vi "SLM_Calibrator_MANUAL.vi"() -> ()   [LabVIEW 2022 SP3]
uses:
  <vilib>/Utility/error.llb/DialogType.ctl
panel:
  out "error out 2":errorcluster
  out "error out":errorcluster
  out "return value":T1={"x"=2592, "y"=1944, "FPS"=20.50524934383202, "Exposure"=70.26569}
  out "available cameras":cluster{string[], string[]}={["U3-368xXLE-M", "U3-38JxXLE-M"], ["4104401787", "4104527767"]}
  in  "Yoffset 2":dbl
  in  "Xoffset 2":dbl
  in  "Yoffset":dbl=-57.0
  in  "Xoffset":dbl=1306.0
  in  "wait time (s)":u32=2
  in  "Tab Control":enum32{"CCD plane", "Plot"}(tab)=enum."Plot"
  in  "FPS":dbl=20.50524934383202
  out "Image Out":T2(plugin-control)
  in  "Exposure":dbl=70.26569
  in  "Camera ID":u16(ring) caption="Camera" items=["U3-368xXLE-M", "U3-38JxXLE-M"]
  out "XY Graph":cluster{dbl, dbl}[](graph)
  out "45º":bool
  out "135º":bool=TRUE
  in  "Analizer":bool=TRUE
  in  "Gradient2":bool
  in  "Gradient1":bool
  out "Yi2":dbl=-234.1726618705036
  in  "Yc2":dbl(slide)=4.136690647482014 scale=0.0..10.0
  in  "Yf2:":dbl(slide)=5.467625899280575 scale=0.0..10.0
  out "Xi2":dbl=82.7639751552795
  in  "Xf2:":dbl(slide)=5.372670807453416 scale=0.0..10.0
  in  "Xc2":dbl(slide)=1.1180124223602483 scale=0.0..10.0
  out "CGH_y\nSLM2":T2(plugin-control)
  in  "Active1":bool=TRUE caption="Hide/Show (Show)"
  in  "Active2":bool=TRUE caption="Hide/Show (Show)"
  in  "STOP":bool caption="Stop (F)"
  out "PHASE":bool
  out "AMP":bool=TRUE
  in  "amp_phase":bool=TRUE
  out "SLM2 2":bool
  out "SLM1":bool=TRUE
  in  "SLMs":bool=TRUE
  in  "Folter to save:":string="IDSfirst"
  out "Images done":dbl(slide) scale=0.0..256.0
  out "Yi1":dbl=-61.63636363636361
  out "Xi1":dbl=1319.9969418960245
  in  "Yf1:":dbl(slide)=-2.1636363636363636 min=-5.0 max=5.0 scale=-5.0..5.0
  in  "Xf1:":dbl(slide)=0.20000000000000018 min=-5.0 max=5.0 scale=-5.0..5.0
  in  "Xc1":dbl(slide)=0.25993883792048944 scale=-5.0..5.0
  in  "Yc1":dbl(slide)=0.30909090909090864 scale=-5.0..5.0
  out "CGH_x\nSLM1":T2(plugin-control)
  in  "Ready?\nCalibrate!":bool caption="Stop (F)"
  # "X:"
  # "Y:"
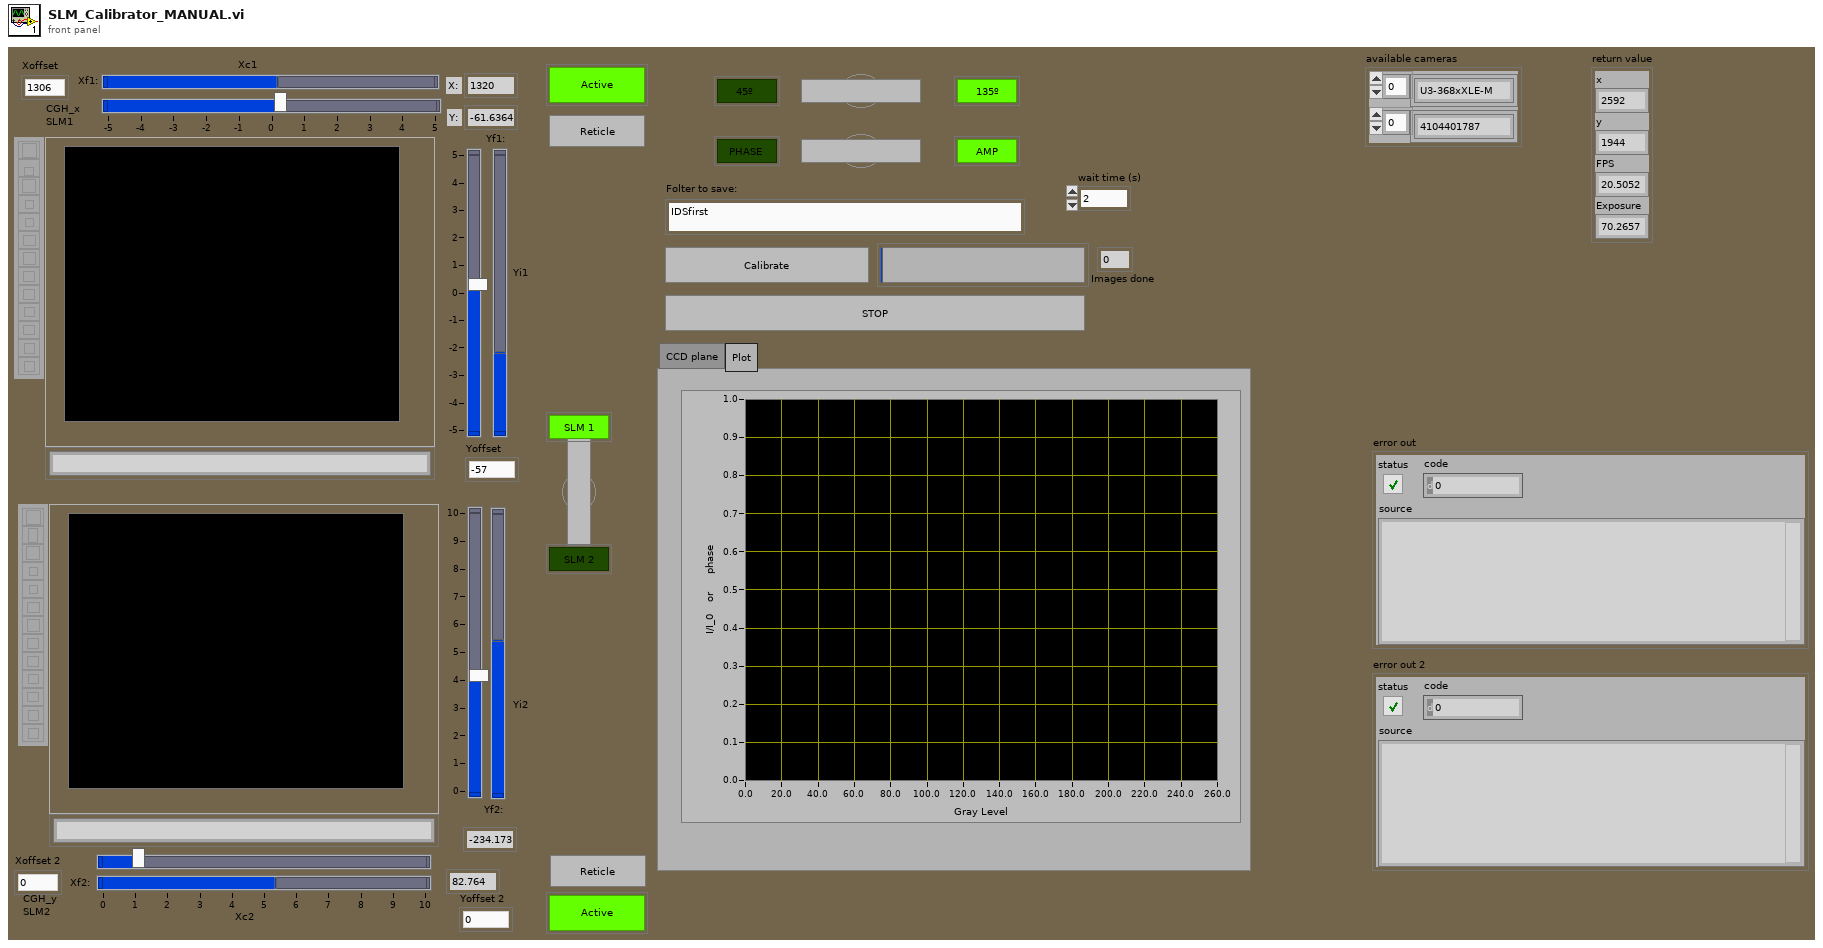
[diagram p1: front panel]
types:
  T1 = cluster{"x":i32, "y":i32, "FPS":dbl, "Exposure":dbl}
  T2 = typedef "IMAQ Image.ctl" = refnum<image>
  T3 = typedef "Image Type" = u32
  T4 = cluster{"Xoffset":dbl, "Yoffset":dbl, "Xc1":dbl, "Yc1":dbl, "Xf1:":dbl, "Yf1:":dbl}
  T5 = cluster{"Xoffset 2":dbl, "Yoffset 2":dbl, "Xc2":dbl, "Yc2":dbl, "Xf2:":dbl, "Yf2:":dbl}
  T6 = typedef "DialogType.ctl" = u16
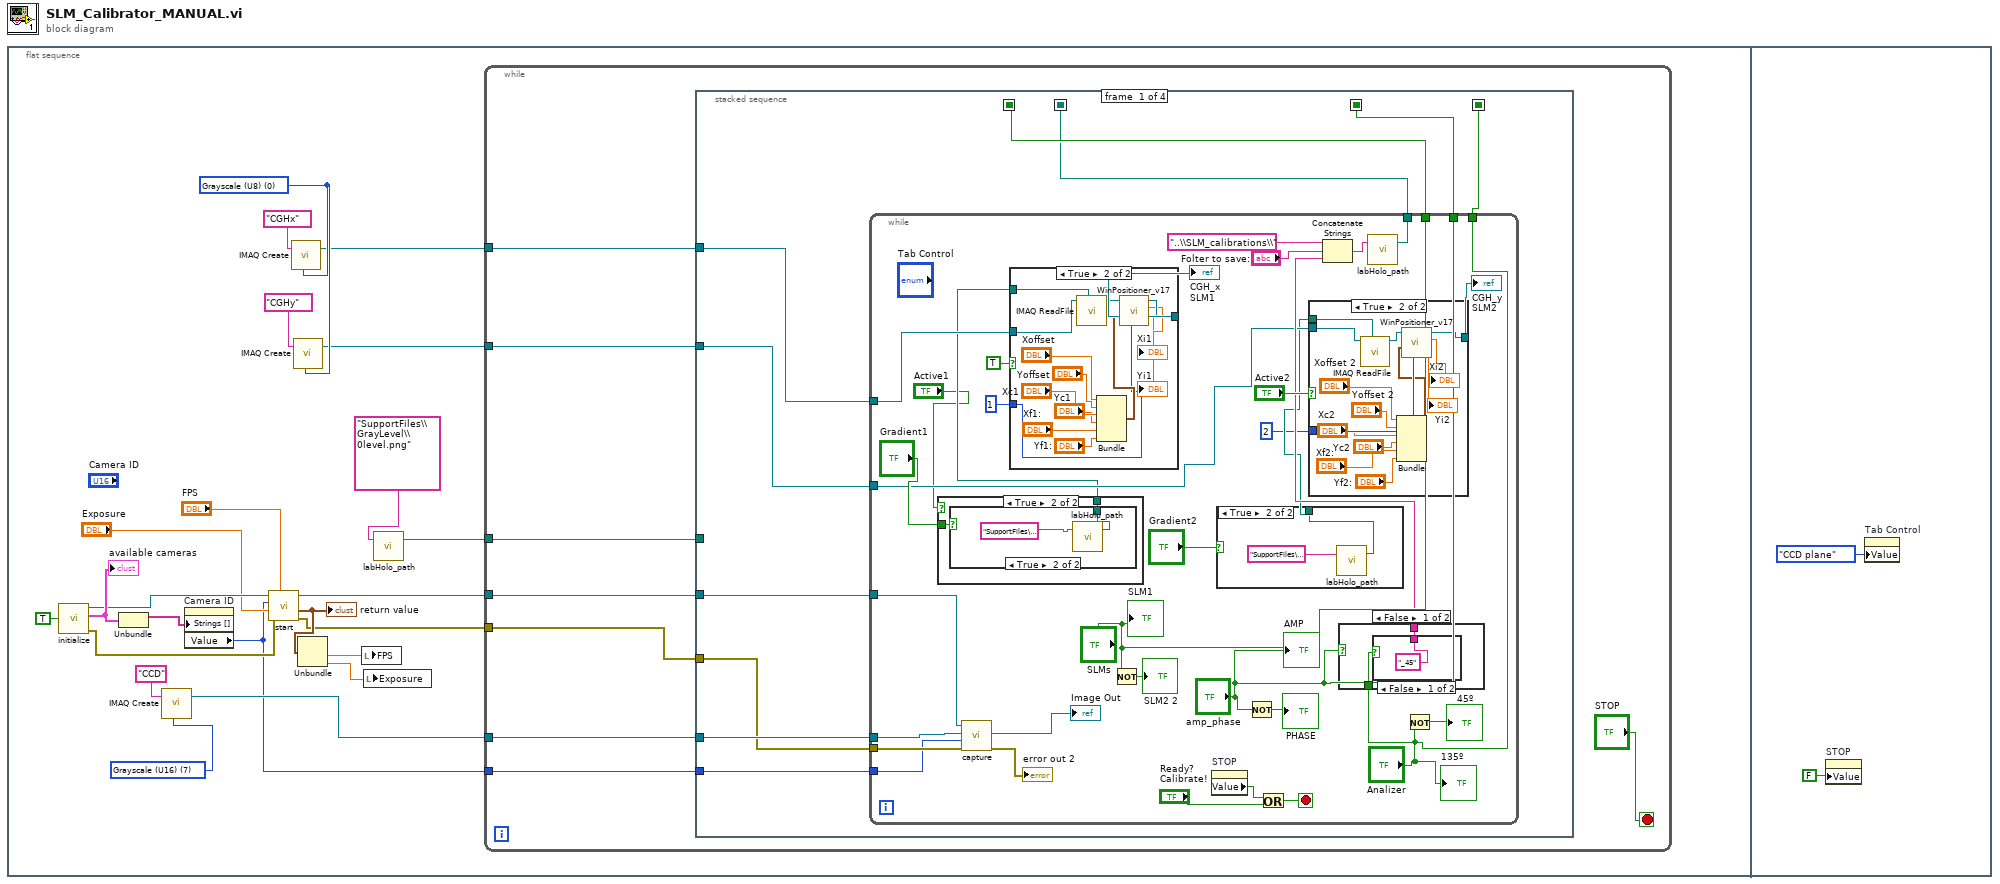
[diagram p0: block diagram]
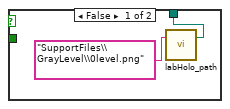
[diagram p2: hidden frame]
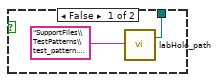
[diagram p3: hidden frame]
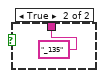
[diagram p4: hidden frame]
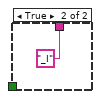
[diagram p5: hidden frame]
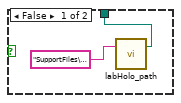
[diagram p6: hidden frame]
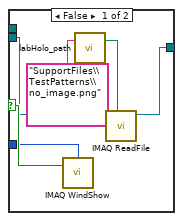
[diagram p7: hidden frame]
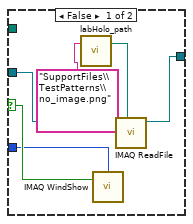
[diagram p8: hidden frame]
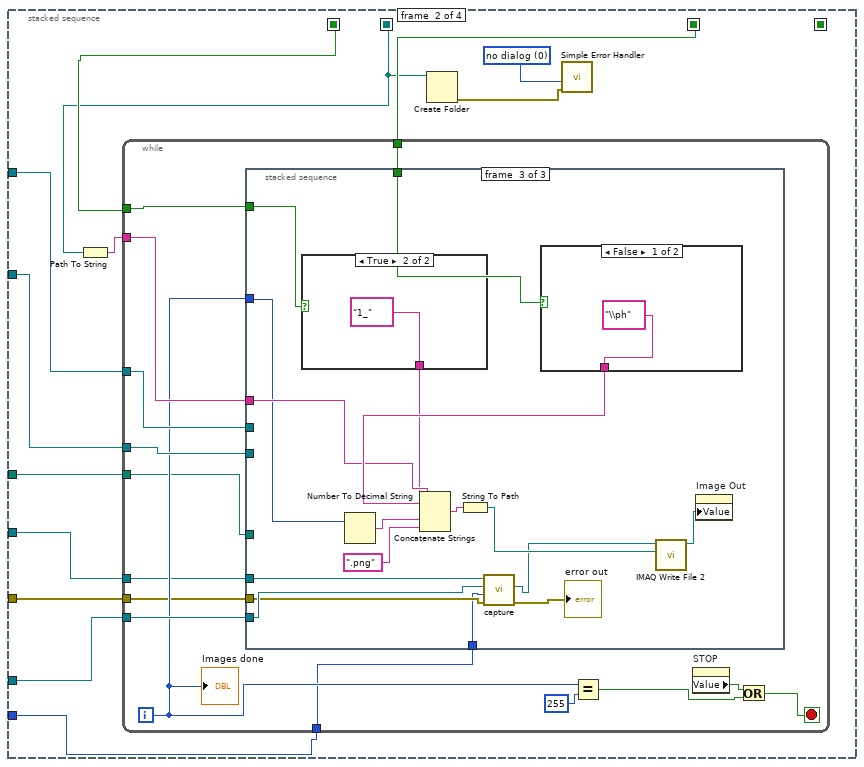
[diagram p9: hidden frame]
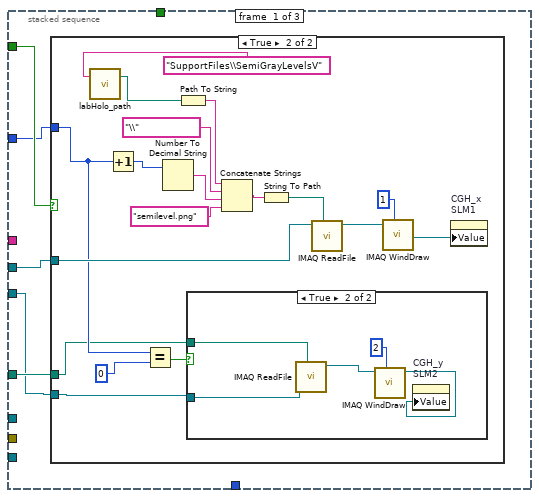
[diagram p10: hidden frame]
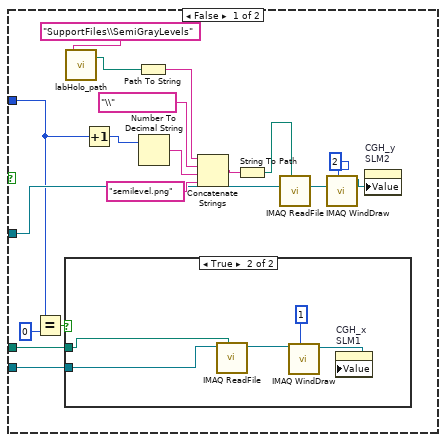
[diagram p11: hidden frame]
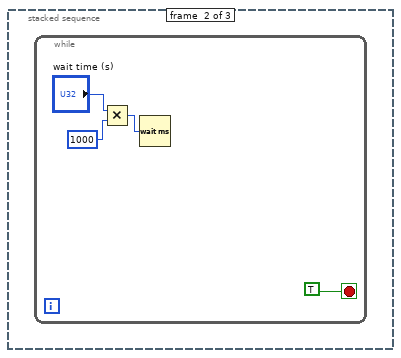
[diagram p14: hidden frame]
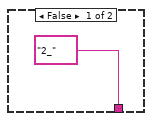
[diagram p15: hidden frame]
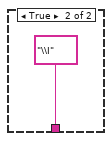
[diagram p16: hidden frame]
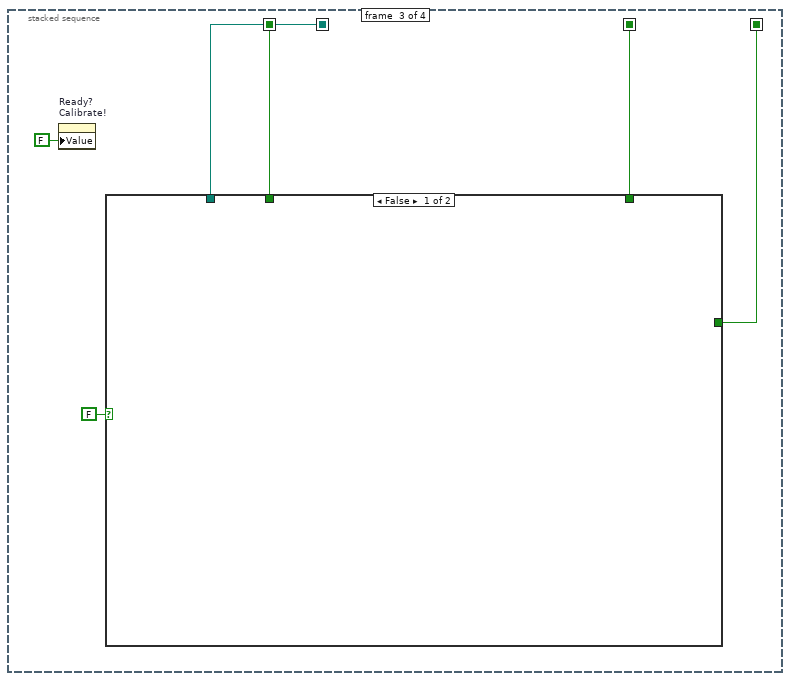
[diagram p17: hidden frame]
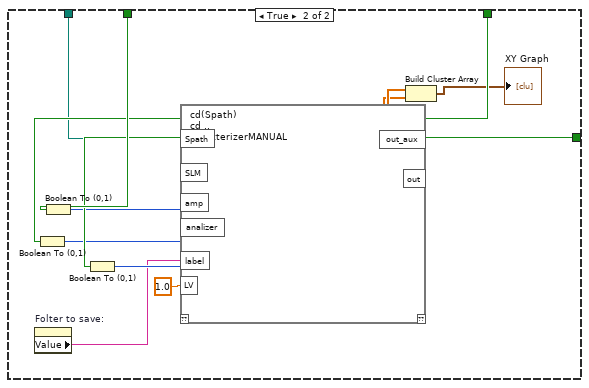
[diagram p18: hidden frame]
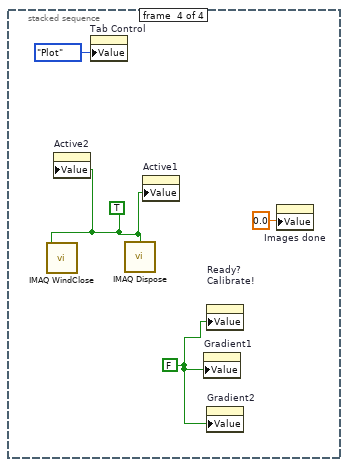
[diagram p19: hidden frame]
diagram:
  n1 = flat-sequence {
    frame #0 {
      w6 = T3 0 items=["Grayscale (U8)", "Grayscale (I16)", "Grayscale (SGL)", "Complex (CSG)", "RGB (U32)", "HSL (U32)", "RGB (U64)", "Grayscale (U16)"] ("Image Type")
      w21 = T3 7 items=["Grayscale (U8)", "Grayscale (I16)", "Grayscale (SGL)", "Complex (CSG)", "RGB (U32)", "HSL (U32)", "RGB (U64)", "Grayscale (U16)"] ("Image Type")
      n2 = call "initialize.vi"("14bits"=TRUE) -> ("session out"=w17:refnum<k35>, "available cameras"=w19:cluster{string[], string[]}, "error out"=w14:errorcluster)  [unwired: 3 in]
      "available cameras" <- w19
      n3 = Unbundle(w19) -> (w18:string[])  [unwired: 1 out]
      n4 = call "IMAQ Create"("Image Name"="CCD", "Image Type"=w21) -> ("New Image"=w20:T2)  [unwired: 3 in, 1 out]
      n5 = property on="Camera ID" class="Ring (strict)"("Strings []"=w18) -> ("Value"=w8:u16)  [unwired: 2 in, 2 out]
      n6 = call "start.vi"("FPS"="FPS", "error in (no error)"=w14, "Exposure (ms)"="Exposure", "Cam id"=w8, "session in"=w17) -> ("error out"=w9:errorcluster, "return value"=w13:T1, "session out"=w10:refnum<k35>)  [unwired: 2 in]
      "return value" <- w13
      n7 = call "IMAQ Create"("Image Name"="CGHx", "Image Type"=w6) -> ("New Image"=w3:T2)  [unwired: 3 in, 1 out]
      n8 = call "IMAQ Create"("Image Name"="CGHy", "Image Type"=w6) -> ("New Image"=w4:T2)  [unwired: 3 in, 1 out]
      n9 = Unbundle(w13) -> ("FPS"=w12:dbl, "Exposure"=w11:dbl)  [unwired: 2 out]
      n10 = local write "FPS"(w12) -> ()
      n11 = local write "Exposure"(w11) -> ()
      n12 = call "labHolo_path.vi"("sub folder or file (str)"="SupportFiles\\GrayLevel\\0level.png" ("name or relative path")) -> ("labHolo path"=w1:path)  [unwired: 1 in, 1 out]
      n13 = while {
        tunnel: w20 -> [w30]
        tunnel: w10 -> [w29]
        tunnel: w9 -> [w28]
        tunnel: w8 -> [w27]
        tunnel: w4 -> [w26]
        tunnel: w3 -> [w25]
        tunnel: w1 -> [w24]
        stop <- "STOP" stop-if-true
        n14 = stacked-sequence {
          seq-local: [w33 _ _ _] -> [_ w138 w239 _]
          seq-local: [w40 _ _ _] -> [_ w140 w241 _]
          seq-local: [w32 _ _ _] -> [_ w141 w240 _]
          seq-local: [w37 _ _ _] -> [_ _ w238 _]
          tunnel: w26 -> [w38 w143 _ _]
          tunnel: w25 -> [w39 w144 _ _]
          tunnel: w30 -> [w41 w139 _ _]
          tunnel: w29 -> [w36 w135 _ _]
          tunnel: w28 -> [w35 w134 _ _]
          tunnel: w27 -> [w34 w132 _ _]
          tunnel: w24 -> [_ w133 _ _]
          frame #0 {
            n15 = while {
              tunnel: w41 -> [w49]
              tunnel: [w42] -> w33
              tunnel: ["amp_phase"] -> w32
              tunnel: ["SLMs"] -> w40
              tunnel: w39 -> [w55]
              tunnel: w38 -> [w57]
              tunnel: ["Analizer"] -> w37
              tunnel: w36 -> [w47]
              tunnel: w35 -> [w46]
              tunnel: w34 -> [w45]
              stop <- w71 stop-if-true
              n16 = case shown="True" "Active1" {
                tunnel: "Gradient1" -> [_ w78]
                tunnel: [w75 w77] -> w54
                frame False {
                  n17 = call "labHolo_path.vi"("sub folder or file (str)"="SupportFiles\\GrayLevel\\0level.png" ("name or relative path")) -> ("labHolo path"=w75:path)  [unwired: 1 in, 1 out]
                }
                frame True {
                  n18 = case shown="True" w78 {
                    tunnel: [w79 w82] -> w77
                    frame False {
                      n19 = call "labHolo_path.vi"("sub folder or file (str)"="SupportFiles\\TestPatterns\\test_pattern.bmp" ("name or relative path")) -> ("labHolo path"=w79:path)  [unwired: 1 in, 1 out]
                    }
                    frame True {
                      n20 = call "labHolo_path.vi"("sub folder or file (str)"="SupportFiles\\TestPatterns\\test_pattern2V.png" ("name or relative path")) -> ("labHolo path"=w82:path)  [unwired: 1 in, 1 out]
                    }
                  }
                }
              }
              n21 = call "capture.vi"("error in (no error)"=w46, "Cam ID"=w45, "Image in"=w49, "session in"=w47) -> ("error out"=→"error out 2":errorcluster, "Image out"=→"Image Out":T2)  [unwired: 3 in, 1 out]
              n22 = case shown="True" TRUE {
                selector: TRUE -> [w117 _]
                tunnel: [w116 w128] -> w68
                tunnel: w55 -> [w115 w131]
                tunnel: w54 -> [_ w130]
                tunnel: 1 ("Window Number (0...15)") -> [w114 w118]
                frame False {
                  n23 = call "labHolo_path.vi"("sub folder or file (str)"="SupportFiles\\TestPatterns\\no_image.png" ("name or relative path")) -> ("labHolo path"=w112:path)  [unwired: 1 in, 1 out]
                  n24 = call "IMAQ WindShow"("Hide/Show (Show)"=w117, "Window Number (0...15)"=w114) -> ()  [unwired: 4 in, 3 out]
                  n25 = call "IMAQ ReadFile"("File Path"=w112, "Image"=w115) -> ("Image Out"=w116:T2)  [unwired: 5 in, 4 out]
                }
                frame True {
                  n26 = call "IMAQ ReadFile"("File Path"=w130, "Image"=w131) -> ("Image Out"=w129:T2)  [unwired: 5 in, 4 out]
                  n27 = Bundle("Xoffset"="Xoffset", "Yoffset"="Yoffset", "Xc1"="Xc1", "Yc1"="Yc1", "Xf1:"="Xf1:", "Yf1:"="Yf1:") -> (w125:T4)  [unwired: 1 in]
                  n28 = call "WinPositioner_v17.vi"("Display (1, 2...)"=w118, "Cluster"=w125, "Image"=w129) -> ("Y position"=→"Yi1":dbl, "X position"=→"Xi1":dbl, "CGH_x"=w128:T2)  [unwired: 6 in]
                }
              }
              "CGH_x\nSLM1" <- w68
              n29 = Not(x="SLMs") -> (.not. x?=→"SLM2 2":bool)
              n30 = property on="STOP" class="Bool (strict)"() -> ("Value"=w70:bool)  [unwired: 2 in, 2 out]
              n31 = case shown="True" "Gradient2" {
                tunnel: [w88 w90] -> w56
                frame False {
                  n32 = call "labHolo_path.vi"("sub folder or file (str)"="SupportFiles\\TestPatterns\\test_pattern.bmp" ("name or relative path")) -> ("labHolo path"=w88:path)  [unwired: 1 in, 1 out]
                }
                frame True {
                  n33 = call "labHolo_path.vi"("sub folder or file (str)"="SupportFiles\\TestPatterns\\test_pattern2.png" ("name or relative path")) -> ("labHolo path"=w90:path)  [unwired: 1 in, 1 out]
                }
              }
              n34 = Not(x="amp_phase") -> (.not. x?=→"PHASE":bool)
              n35 = Or(x=w70, y="Ready?\nCalibrate!") -> (x .or. y?=w71:bool)
              n36 = case shown="True" "Active2" {
                selector: "Active2" -> [w97 _]
                tunnel: [w95 w106] -> w66
                tunnel: w57 -> [w96 w109]
                tunnel: w56 -> [_ w108]
                tunnel: 2 ("Window Number (0...15)") -> [w94 w107]
                frame False {
                  n37 = call "IMAQ WindShow"("Hide/Show (Show)"=w97, "Window Number (0...15)"=w94) -> ()  [unwired: 4 in, 3 out]
                  n38 = call "labHolo_path.vi"("sub folder or file (str)"="SupportFiles\\TestPatterns\\no_image.png" ("name or relative path")) -> ("labHolo path"=w92:path)  [unwired: 1 in, 1 out]
                  n39 = call "IMAQ ReadFile"("File Path"=w92, "Image"=w96) -> ("Image Out"=w95:T2)  [unwired: 5 in, 4 out]
                }
                frame True {
                  n40 = call "IMAQ ReadFile"("File Path"=w108, "Image"=w109) -> ("Image Out"=w105:T2)  [unwired: 5 in, 4 out]
                  n41 = Bundle("Xoffset 2"="Xoffset 2", "Yoffset 2"="Yoffset 2", "Xc2"="Xc2", "Yc2"="Yc2", "Xf2:"="Xf2:", "Yf2:"="Yf2:") -> (w98:T5)  [unwired: 1 in]
                  n42 = call "WinPositioner_v17.vi"("Display (1, 2...)"=w107, "Cluster"=w98, "Image"=w105) -> ("Y position"=→"Yi2":dbl, "X position"=→"Xi2":dbl, "CGH_x"=w106:T2)  [unwired: 6 in]
                }
              }
              "CGH_y\nSLM2" <- w66
              n43 = case shown="False" "amp_phase" {
                tunnel: "Analizer" -> [w84 _]
                tunnel: [w83 "_I"] -> w59
                frame False {
                  n44 = case shown="False" w84 {
                    tunnel: ["_45" "_135"] -> w83
                    frame False {
                    }
                    frame True {
                    }
                  }
                }
                frame True {
                }
              }
              n45 = Concatenate Strings("..\\SLM_calibrations\\" ("string"), "Folter to save:", w59) -> (w43:string)
              n46 = call "labHolo_path.vi"("sub folder or file (str)"=w43) -> ("labHolo path"=w42:path)  [unwired: 1 in, 1 out]
              n47 = Not(x="Analizer") -> (.not. x?=→"45º":bool)
              "SLM1" <- "SLMs"
              "AMP" <- "amp_phase"
              "135º" <- "Analizer"
            }
          }
          frame #1 {
            w137 = T6 0 items=["no dialog", "OK message", "continue or stop message", "OK message + warnings", "continue/stop + warnings"] ("type of dialog (OK msg:1)")
            n48 = Path To String(path=w138) -> (string=w142:string)
            n49 = while {
              tunnel: w144 -> [w156]
              tunnel: w143 -> [w158]
              tunnel: w140 -> [w159]
              tunnel: w142 -> [w157]
              tunnel: w141 -> [w155]
              tunnel: w139 -> [w154]
              tunnel: w135 -> [w148]
              tunnel: w134 -> [w147]
              tunnel: w133 -> [w146]
              tunnel: w132 -> [w145]
              i -> [w151]
              stop <- w149 stop-if-true
              n50 = stacked-sequence {
                tunnel: w151 -> [w160 _ w218]
                tunnel: w157 -> [_ _ w227]
                tunnel: w159 -> [w161 _ w225]
                tunnel: w156 -> [w164 _ _]
                tunnel: w158 -> [w162 _ _]
                tunnel: w155 -> [_ _ w226]
                tunnel: w154 -> [_ _ w220]
                tunnel: w146 -> [w163 _ _]
                tunnel: w148 -> [_ _ w221]
                tunnel: w147 -> [_ _ w217]
                tunnel: w145 -> [_ _ w215]
                frame #0 {
                  n51 = case shown="True" w161 {
                    tunnel: w162 -> [w181 w196]
                    tunnel: w160 -> [w170 w192]
                    tunnel: w164 -> [w174 w195]
                    tunnel: w163 -> [w168 w190]
                    frame False {
                      n52 = Equal?(x=w170, y=0) -> (x = y?=w171:bool)
                      n53 = case shown="True" w171 {
                        tunnel: w181 -> [_ w186]
                        tunnel: w168 -> [_ w183]
                        frame False {
                        }
                        frame True {
                          n54 = call "IMAQ ReadFile"("File Path"=w183, "Image"=w186) -> ("Image Out"=w187:T2)  [unwired: 5 in, 4 out]
                          n55 = call "IMAQ WindDraw"("Window Number (0...15)"=1, "Image"=w187) -> ("Image Out (duplicate)"=w185:T2)  [unwired: 8 in, 1 out]
                          n56 = property on="CGH_x\nSLM1" class="ImageControl"("Value"=w185) -> ()  [unwired: 2 in, 2 out]
                        }
                      }
                      n57 = call "labHolo_path.vi"("sub folder or file (str)"="SupportFiles\\SemiGrayLevels" ("name or relative path")) -> ("labHolo path"=w166:path)  [unwired: 1 in, 1 out]
                      n58 = Increment(x=w170) -> (x+1=w177:i32)
                      n59 = Path To String(path=w166) -> (string=w179:string)
                      n60 = Number To Decimal String(number=w177) -> (decimal integer string=w178:string)  [unwired: 1 in]
                      n61 = Concatenate Strings(w179, "\\", w178, "semilevel.png") -> (w175:string)
                      n62 = String To Path(string=w175) -> (path=w173:path)
                      n63 = call "IMAQ ReadFile"("File Path"=w173, "Image"=w174) -> ("Image Out"=w182:T2)  [unwired: 5 in, 4 out]
                      n64 = call "IMAQ WindDraw"("Window Number (0...15)"=2, "Image"=w182) -> ("Image Out (duplicate)"=w167:T2)  [unwired: 8 in, 1 out]
                      n65 = property on="CGH_y\nSLM2" class="ImageControl"("Value"=w167) -> ()  [unwired: 2 in, 2 out]
                    }
                    frame True {
                      n66 = call "labHolo_path.vi"("sub folder or file (str)"="SupportFiles\\SemiGrayLevelsV" ("name or relative path")) -> ("labHolo path"=w188:path)  [unwired: 1 in, 1 out]
                      n67 = Increment(x=w192) -> (x+1=w199:i32)
                      n68 = Equal?(x=w192, y=0) -> (x = y?=w193:bool)
                      n69 = Number To Decimal String(number=w199) -> (decimal integer string=w200:string)  [unwired: 1 in]
                      n70 = Path To String(path=w188) -> (string=w201:string)
                      n71 = case shown="True" w193 {
                        tunnel: w196 -> [_ w208]
                        tunnel: w190 -> [_ w207]
                        frame False {
                        }
                        frame True {
                          n72 = call "IMAQ ReadFile"("File Path"=w207, "Image"=w208) -> ("Image Out"=w210:T2)  [unwired: 5 in, 4 out]
                          n73 = call "IMAQ WindDraw"("Window Number (0...15)"=2, "Image"=w210) -> ("Image Out (duplicate)"=w206:T2)  [unwired: 8 in, 1 out]
                          n74 = property on="CGH_y\nSLM2" class="ImageControl"("Value"=w206) -> ()  [unwired: 2 in, 2 out]
                        }
                      }
                      n75 = Concatenate Strings(w201, "\\", w200, "semilevel.png") -> (w197:string)
                      n76 = String To Path(string=w197) -> (path=w194:path)
                      n77 = call "IMAQ ReadFile"("File Path"=w194, "Image"=w195) -> ("Image Out"=w205:T2)  [unwired: 5 in, 4 out]
                      n78 = call "IMAQ WindDraw"("Window Number (0...15)"=1, "Image"=w205) -> ("Image Out (duplicate)"=w204:T2)  [unwired: 8 in, 1 out]
                      n79 = property on="CGH_x\nSLM1" class="ImageControl"("Value"=w204) -> ()  [unwired: 2 in, 2 out]
                    }
                  }
                }
                frame #1 {
                  n80 = while {
                    stop <- TRUE stop-if-true
                    n81 = Multiply(x="wait time (s)", y=u32 1000 ("milliseconds to wait 2")) -> (x*y=w211:u32)
                    n82 = Wait (ms)(milliseconds to wait=w211) -> ()  [unwired: 1 out]
                  }
                }
                frame #2 {
                  n83 = case shown="True" w225 {
                    tunnel: ["2_" "1_"] -> w224
                    frame False {
                    }
                    frame True {
                    }
                  }
                  n84 = Number To Decimal String(number=w218) -> (decimal integer string=w223:string)  [unwired: 1 in]
                  n85 = call "capture.vi"("error in (no error)"=w217, "Cam ID"=w215, "Image in"=w220, "session in"=w221) -> ("error out"=→"error out":errorcluster, "Image out"=w219:T2)  [unwired: 3 in, 1 out]
                  n86 = case shown="False" w226 {
                    tunnel: ["\\ph" "\\I"] -> w230
                    frame False {
                    }
                    frame True {
                    }
                  }
                  n87 = Concatenate Strings(w227, w230, w224, w223, ".png") -> (w229:string)
                  n88 = String To Path(string=w229) -> (path=w228:path)
                  n89 = call-poly "IMAQ Write File 2"("File Path"=w228, "Image"=w219) -> ("Image Out (duplicate)"=w231:T2)  [unwired: 8 in, 1 out]
                  n90 = property on="Image Out" class="ImageControl"("Value"=w231) -> ()  [unwired: 2 in, 2 out]
                }
              }
              n91 = Equal?(x=w151, y=255) -> (x = y?=w150:bool)
              n92 = property on="STOP" class="Bool (strict)"() -> ("Value"=w153:bool)  [unwired: 2 in, 2 out]
              n93 = Or(x=w153, y=w150) -> (x .or. y?=w149:bool)
              "Images done" <- w151
            }
            n94 = Create Folder(path (use dialog)=w138) -> (error out=w136:errorcluster)  [unwired: 2 in, 2 out]
            n95 = call <vilib>:"Simple Error Handler.vi"("type of dialog (OK msg:1)"=w137, "error in (no error)"=w136) -> ()  [unwired: 3 in, 5 out]
          }
          frame #2 {
            n96 = property on="Ready?\nCalibrate!" class="Bool (strict)"("Value"=FALSE ("Ready?\nCalibrate!")) -> ()  [unwired: 2 in, 2 out]
            n97 = case shown="False" FALSE {
              tunnel: w241 -> [_ w253]
              tunnel: w240 -> [_ w252]
              tunnel: w239 -> [_ w247]
              tunnel: w238 -> [_ w251]
              frame False {
              }
              frame True {
                n98 = property on="Folter to save:" class="Str"() -> ("Value"=w243:string)  [unwired: 2 in, 2 out]
                n99 = Boolean To (0,1)(Boolean=w252) -> (0, 1=w249:i16)
                n100 = Boolean To (0,1)(Boolean=w253) -> (0, 1=w250:i16)
                n101 = Boolean To (0,1)(Boolean=w251) -> (0, 1=w248:i16)
                n102 = script code="cd(Spath)\ncd ..\ncaracterizerMANUAL"("SLM"=w250, "amp"=w249, "Spath"=w247, "analizer"=w248, "label"=w243, "LV"=1.0 ("Real")) -> ("out"=w245:dbl[], "out_aux"=w246:dbl[])  [unwired: 1 in, 1 out]
                n103 = Build Cluster Array(w246, w245) -> (→"XY Graph":cluster{dbl, dbl}[])
              }
            }
          }
          frame #3 {
            w255 = TRUE ("Close All Windows (False)")
            w256 = FALSE ("Ready?\nCalibrate!")
            n104 = call "IMAQ WindClose"("Close All Windows (False)"=w255) -> ()  [unwired: 5 in, 1 out]
            n105 = property on="Active2" class="Bool (strict)"("Value"=w255) -> ()  [unwired: 2 in, 2 out]
            n106 = property on="Tab Control" class="TabCtl (strict)"("Value"=enum32{"CCD plane", "Plot"}."Plot" ("Tab Control")) -> ()  [unwired: 2 in, 2 out]
            n107 = call "IMAQ Dispose"("All Images? (No)"=w255) -> ()  [unwired: 5 in, 1 out]
            n108 = property on="Active1" class="Bool (strict)"("Value"=w255) -> ()  [unwired: 2 in, 2 out]
            n109 = property on="Gradient1" class="Bool (strict)"("Value"=w256) -> ()  [unwired: 2 in, 2 out]
            n110 = property on="Ready?\nCalibrate!" class="Bool (strict)"("Value"=w256) -> ()  [unwired: 2 in, 2 out]
            n111 = property on="Gradient2" class="Bool (strict)"("Value"=w256) -> ()  [unwired: 2 in, 2 out]
            n112 = property on="Images done" class="Slide (strict)"("Value"=0.0 ("Images done")) -> ()  [unwired: 2 in, 2 out]
          }
        }
      }
    }
    frame #1 {
      n113 = property on="STOP" class="Bool (strict)"("Value"=FALSE ("STOP")) -> ()  [unwired: 2 in, 2 out]
      n114 = property on="Tab Control" class="TabCtl (strict)"("Value"=enum32{"CCD plane", "Plot"}."CCD plane" ("Tab Control")) -> ()  [unwired: 2 in, 2 out]
    }
  }
